vi "AdorkableWatchDog_sln.vi"() -> ()   [LabVIEW 2014]
panel:
  in  "Stop Button":bool
  out "Functioning?":bool
  out "InstrumentRunning?":bool
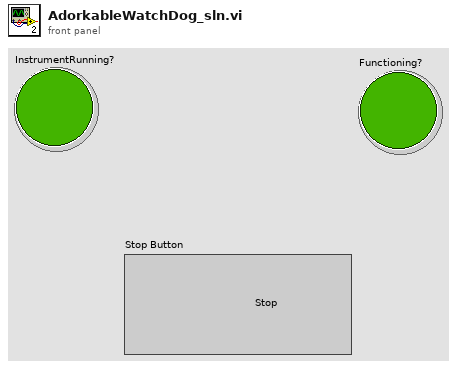
[diagram p1: front panel]
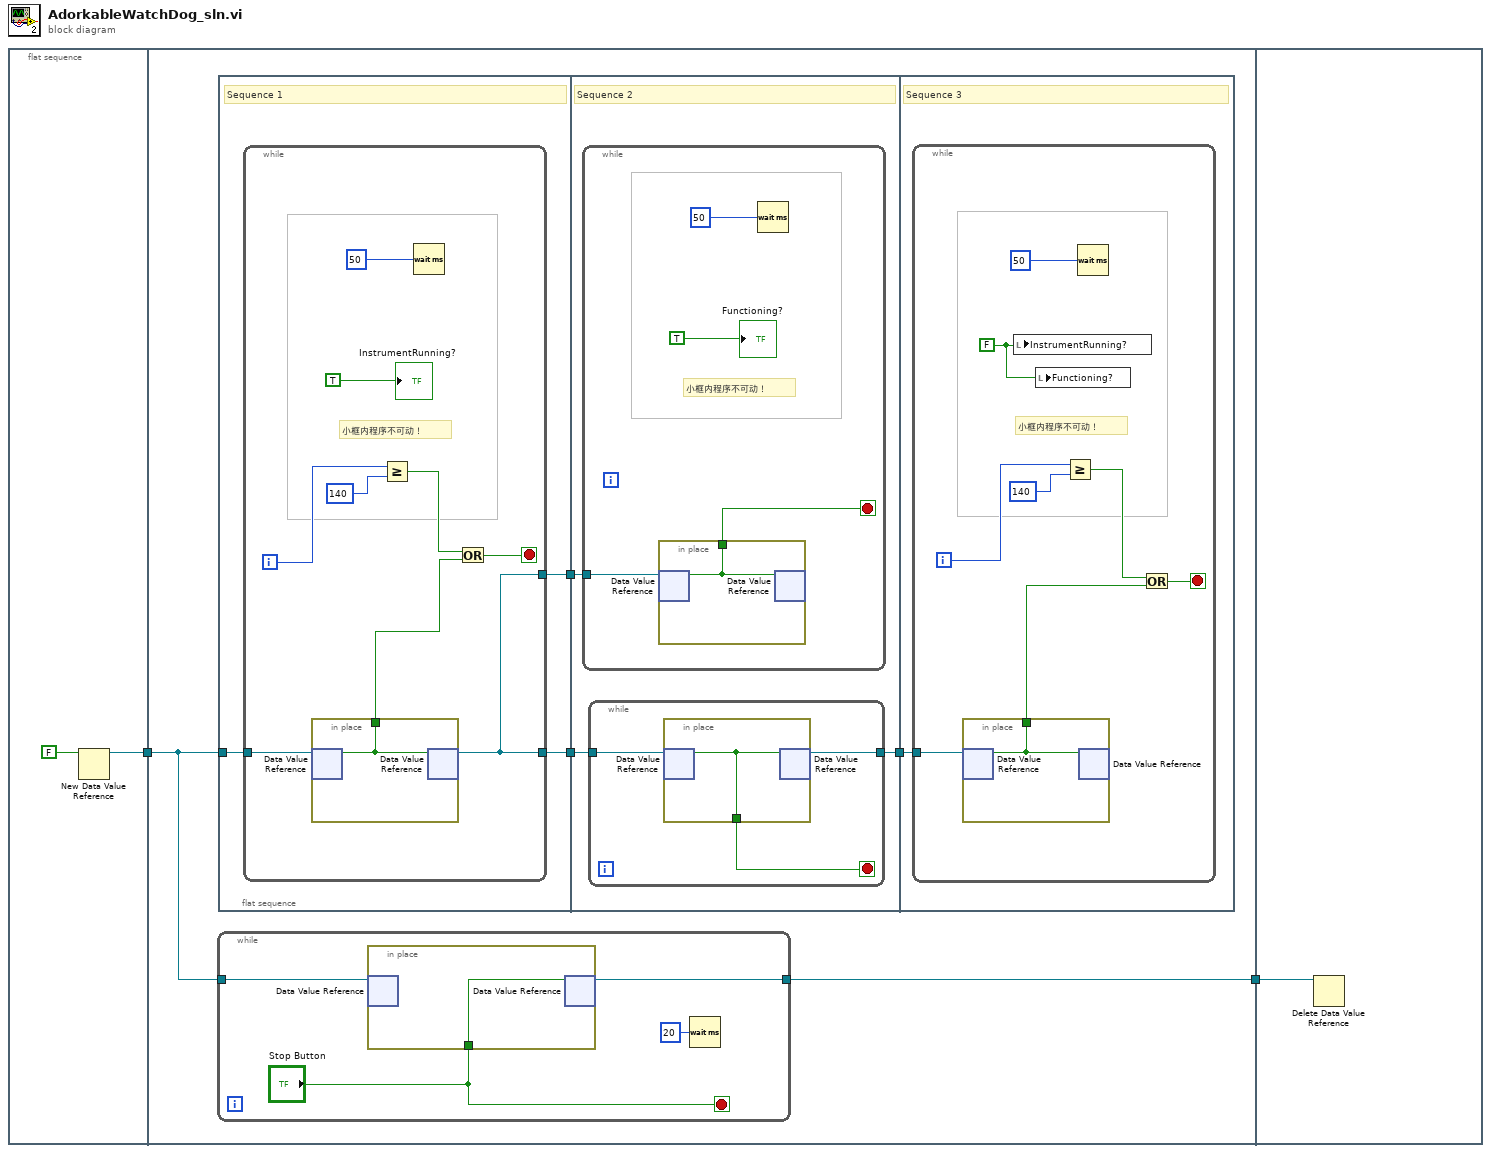
[diagram p0: block diagram]
diagram:
  n1 = flat-sequence {
    tunnel: [w3] -> w2
    tunnel: w2 -> [w9]
    tunnel: [w8] -> w1
    tunnel: w1 -> [w50]
    frame #0 {
      n2 = New Data Value Reference(data value=FALSE) -> (data value reference=w3:refnum<data-value>)  [unwired: 1 in, 1 out]
    }
    frame #1 {
      n3 = while {
        tunnel: w9 -> [w12]
        tunnel: [w11] -> w8
        stop <- "Stop Button" stop-if-true
        n4 = in-place {
          in-place-border: "Stop Button" -> [w14]
          n5 = in-place-dvr #1(w12) -> ()  [unwired: 2 out]
          n6 = in-place-dvr #1(w14) -> (w11:refnum<data-value>)  [unwired: 1 out]
        }
        n7 = Wait (ms)(milliseconds to wait=u32 20) -> ()  [unwired: 1 out]
      }
      n8 = flat-sequence {
        tunnel: w9 -> [w17]
        tunnel: [w16] -> w7
        tunnel: [w15] -> w6
        tunnel: w7 -> [w30]
        tunnel: w6 -> [w29]
        tunnel: [w28] -> w5
        tunnel: w5 -> [w40]
        frame #0 {
          # "Sequence 1"
          n9 = while {
            tunnel: w17 -> [w20]
            tunnel: [w18] -> w16
            tunnel: [w18] -> w15
            i -> [w24]
            stop <- w21 stop-if-true
            # "小框内程序不可动！"
            n10 = in-place {
              in-place-border: [w27] -> w19
              n11 = in-place-dvr #2(w20) -> (w27:bool)  [unwired: 1 out]
              n12 = in-place-dvr #2(w27) -> (w18:refnum<data-value>)  [unwired: 1 out]
            }
            n13 = Greater Or Equal?(x=w24, y=140) -> (x >= y?=w22:bool)
            n14 = Wait (ms)(milliseconds to wait=u32 50) -> ()  [unwired: 1 out]
            n15 = Or(x=w22, y=w19) -> (x .or. y?=w21:bool)
            "InstrumentRunning?" <- TRUE ("InstrumentRunning?")
          }
        }
        frame #1 {
          # "Sequence 2"
          n16 = while {
            tunnel: w29 -> [w36]
            stop <- w35 stop-if-true
            # "小框内程序不可动！"
            n17 = in-place {
              in-place-border: [w39] -> w35
              n18 = in-place-dvr #3(w36) -> (w39:bool)  [unwired: 1 out]
              n19 = in-place-dvr #3(w39) -> ()  [unwired: 2 out]
            }
            n20 = Wait (ms)(milliseconds to wait=u32 50) -> ()  [unwired: 1 out]
            "Functioning?" <- TRUE ("InstrumentRunning?")
          }
          n21 = while {
            tunnel: w30 -> [w33]
            tunnel: [w31] -> w28
            stop <- w32 stop-if-true
            n22 = in-place {
              in-place-border: [w34] -> w32
              n23 = in-place-dvr #4(w33) -> (w34:bool)  [unwired: 1 out]
              n24 = in-place-dvr #4(w34) -> (w31:refnum<data-value>)  [unwired: 1 out]
            }
          }
        }
        frame #2 {
          # "Sequence 3"
          n25 = while {
            tunnel: w40 -> [w42]
            i -> [w45]
            stop <- w44 stop-if-true
            w47 = FALSE ("InstrumentRunning?")
            # "小框内程序不可动！"
            n26 = in-place {
              in-place-border: [w49] -> w41
              n27 = in-place-dvr #5(w42) -> (w49:bool)  [unwired: 1 out]
              n28 = in-place-dvr #5(w49) -> ()  [unwired: 2 out]
            }
            n29 = local write "InstrumentRunning?"(w47) -> ()
            n30 = local write "Functioning?"(w47) -> ()
            n31 = Greater Or Equal?(x=w45, y=140) -> (x >= y?=w43:bool)
            n32 = Wait (ms)(milliseconds to wait=u32 50) -> ()  [unwired: 1 out]
            n33 = Or(x=w43, y=w41) -> (x .or. y?=w44:bool)
          }
        }
      }
    }
    frame #2 {
      n34 = Delete Data Value Reference(data value reference=w50) -> ()  [unwired: 1 in, 2 out]
    }
  }
